vi "统计合格数.vi"(10 "测试时间":string) -> (3 "Rows Fetched":i32)   [LabVIEW 2014]
panel:
  out "Data":string[][](array[string])
  out "error out":errorcluster
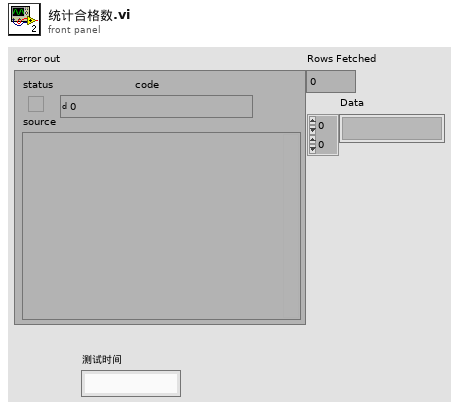
[diagram p1: front panel]
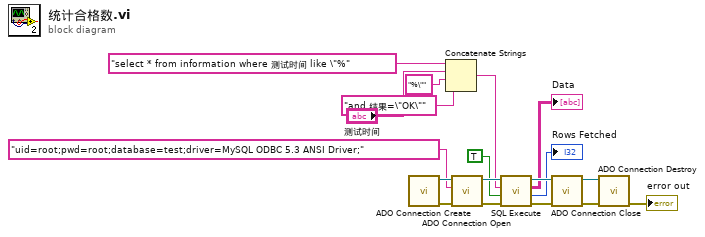
[diagram p0: block diagram]
diagram:
  n1 = call "ADO Connection Create.vi"() -> ("error out"=w17:errorcluster, "ADODB._Connection Out"=w18:refnum<k7>)  [unwired: 10 in]
  n2 = Concatenate Strings("select * from information where 测试时间 like \"%" ("Command Text"), "测试时间", "%\"" ("Command Text"), "and 结果=\"OK\"" ("字符串")) -> (w2:string)
  n3 = call "ADO Connection Open.vi"("error in (no error)"=w17, "ConnectionString"="uid=root;pwd=root;database=test;driver=MySQL ODBC 5.3 ANSI Driver;", "ADODB._Connection In"=w18) -> ("error out"=w15:errorcluster, "ADODB._Connection Out"=w16:refnum<k7>)  [unwired: 7 in]
  n4 = call "SQL Execute.vi"("error in (no error)"=w15, "Return Data (T)"=TRUE, "Command Text"=w2, "ADODB._Connection In"=w16) -> ("error out"=w13:errorcluster, "Rows Fetched"=→"Rows Fetched":i32, "Data"=→"Data":string[][], "ADODB._Connection Out"=w14:refnum<k7>)  [unwired: 4 in]
  n5 = call "ADO Connection Close.vi"("error in (no error)"=w13, "ADODB._Connection In"=w14) -> ("error out"=w11:errorcluster, "ADODB._Connection Out"=w12:refnum<k7>)  [unwired: 8 in]
  n6 = call "ADO Connection Destroy.vi"("error in (no error)"=w11, "ADODB._Connection In"=w12) -> ("error out"=→"error out":errorcluster)  [unwired: 9 in]
